vi "5.vi"   [LabVIEW 2017]
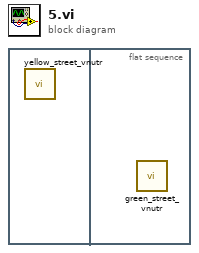
[diagram p0: block diagram]
diagram:
  n1 = flat-sequence {
    frame #0 {
      n2 = call "yellow_street_vnutr.vi"() -> ()  [unwired: 12 in]
    }
    frame #1 {
      n3 = call "green_street_vnutr.vi"() -> ()  [unwired: 12 in]
    }
  }
